vi "rspvtd_Receive System Properties.vi"(8 "error in":errorcluster, 11 "Data in":variant) -> (0 "error out":errorcluster, 3 "Data out":T1 {"System Health Data"."Hard Drive Space Used (%)" scale=0.0..100.0})   [LabVIEW 2017, in "RT System Monitor.lvclass"]
doc: "This VI converts variant data contained in the associated <b>Public API Response</b> message to its correct data type.\n---"
uses:
  RT System Monitor.lvclass
  rsp_Receive System Properties.ctl
  Shared/System Health Data.ctl
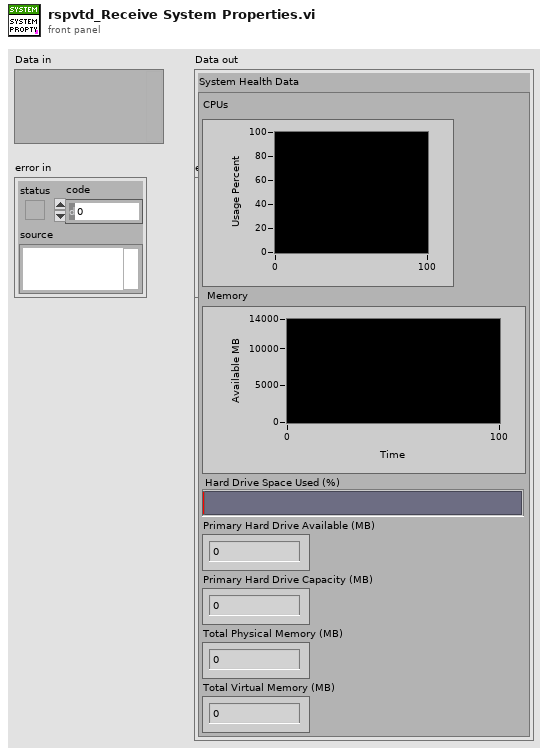
[diagram p1: front panel]
types:
  T1 = typedef "RT System Monitor.lvclass/rsp_Receive System Properties.ctl" = cluster{"System Health Data":T2}
  T2 = typedef "System Health Data.ctl" = cluster{"CPUs":u32[][], "Memory":dbl[][], "Hard Drive Space Used (%)":dbl, "Primary Hard Drive Available (MB)":dbl, "Primary Hard Drive Capacity (MB)":u32, "Total Physical Memory (MB)":u32, "Total Virtual Memory (MB)":u32}
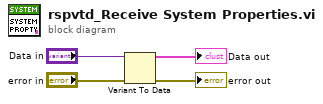
[diagram p0: block diagram]
diagram:
  n1 = Variant To Data(error in="error in", Variant="Data in") -> (data=→"Data out":T1, error out=→"error out":errorcluster)  [unwired: 1 in]
